vi "VISA status.vi"(8 "error in (no error)":errorcluster, 11 "Cobolt in":refnum<class "Cobolt.lvclass">) -> (0 "error out":errorcluster, 3 "Cobolt out":refnum<class "Cobolt.lvclass">)   [LabVIEW 2012, in "Cobolt.lvclass"]
uses:
  Cobolt.lvclass
  Cobolt.lvclass/Cobolt.ctl
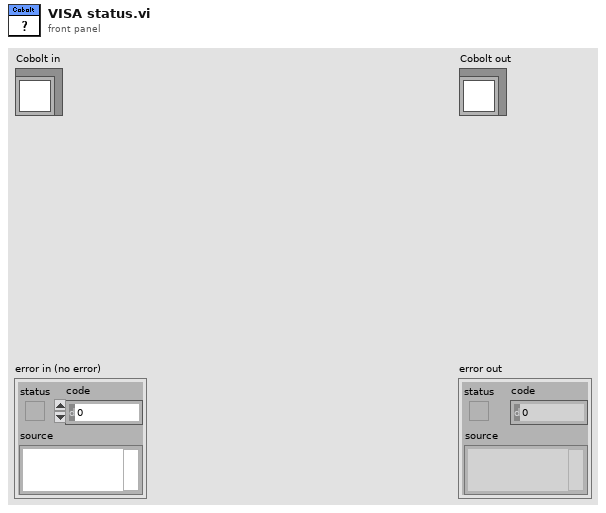
[diagram p1: front panel]
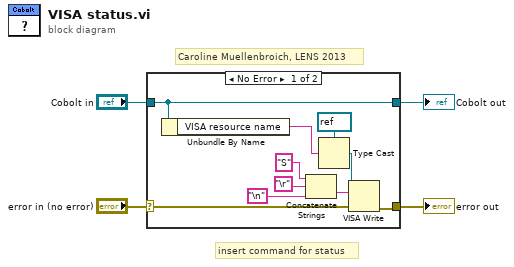
[diagram p0: block diagram]
diagram:
  # "insert command for status"
  # "Caroline Muellenbroich, LENS 2013"
  n1 = case shown="No Error" "error in (no error)" {
    selector: "error in (no error)" -> [w6 w16]
    tunnel: [w5 w16] -> w3
    tunnel: [w9 w15] -> w1
    tunnel: "Cobolt in" -> [w9 w15]
    frame No Error {
      n2 = Unbundle By Name(w9) -> ("VISA resource name"=w8:string)
      n3 = Concatenate Strings("S" ("string"), "\r", "\n") -> (w11:string)
      n4 = Type Cast(type=refnum<visa-resource-name> refnum ("VISA resource name"), x=w8) -> (*(type *) &x=w12:refnum<visa-resource-name>)
      n5 = VISA Write(VISA resource name=w12, write buffer=w11, error in (no error)=w6) -> (error out=w5:errorcluster)  [unwired: 2 out]
    }
    frame Error {
    }
  }
  "error out" <- w3
  "Cobolt out" <- w1
